vi "Remove Actor from DAQ Registry.vi"(8 "error in (no error)":errorcluster, 10 "specific class reference":refnum<class "DAQ Actor.lvclass">, 11 "FP Controls in":refnum<class "FP Controls.lvclass">) -> (0 "error out":errorcluster, 3 "FP Controls out":refnum<class "FP Controls.lvclass">)   [LabVIEW 2018, in "Configuration Grandmaster.lvlib" / "FP Controls.lvclass"]
uses:
  FP Controls.lvclass
  Data Acquisition/Class DAQ Actor/DAQ Actor.lvclass
  FP Controls.lvclass/FP Controls.ctl
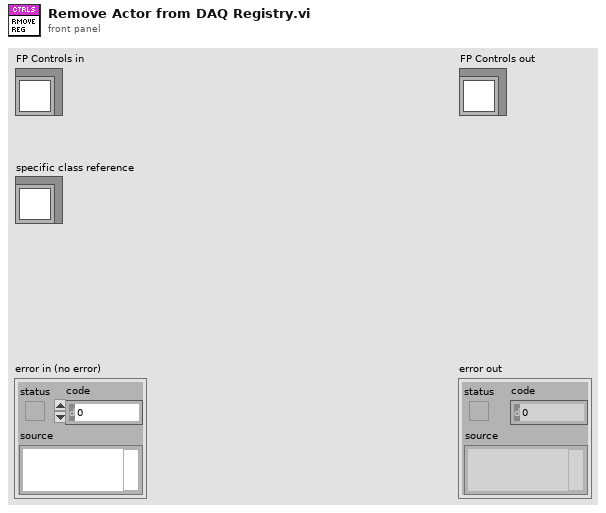
[diagram p1: front panel]
types:
  T1 = typedef "TE_Designator.ctl" = enum16{"High Speed", "Low Speed"}
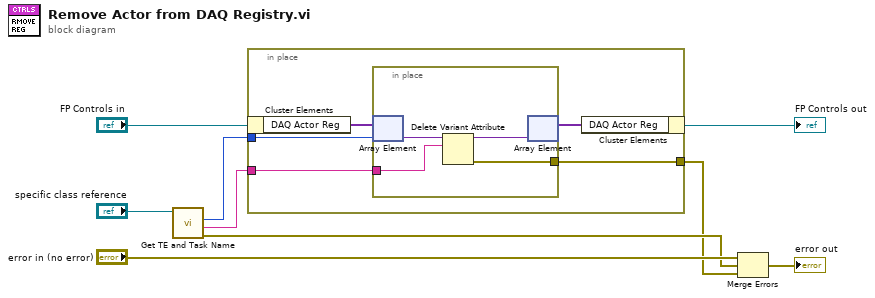
[diagram p0: block diagram]
diagram:
  n1 = call "Get TE and Task Name.vi"("DAQ Actor in"="specific class reference") -> ("error out"=w3:errorcluster, "Task Name"=w5:string, "TimingEngine"=w6:T1)  [unwired: 7 in, 1 out]
  n2 = in-place {
    in-place-border: w6 -> [w13]
    in-place-border: w5 -> [w11]
    in-place-border: [w10] -> w2
    n3 = in-place-cluster #1("FP Controls in") -> ("DAQ Actor Reg"=w14:variant[])
    n4 = in-place {
      in-place-border: w11 -> [w16]
      in-place-border: [w15] -> w10
      n5 = in-place-array #2(w14, w13) -> (w18:variant)
      n6 = Delete Variant Attribute(6:w16, 7:w18) -> (0:w15:errorcluster, 3:w17:variant)  [unwired: 1 in, 1 out]
      n7 = in-place-array #2(w17) -> (w12:variant[])  [unwired: 1 out]
    }
    n8 = in-place-cluster #1("DAQ Actor Reg"=w12) -> (→"FP Controls out":refnum<class "FP Controls.lvclass">)
  }
  n9 = Merge Errors("error in (no error)", w3, w2) -> (→"error out":errorcluster)
